vi "Name.vi"(8 "error in (no error)":errorcluster, 11 "object in":refnum<class "execute_request Message.lvclass">) -> (0 "error out":errorcluster, 2 "Name":string, 3 "object out":refnum<class "execute_request Message.lvclass">)   [LabVIEW 2018, in "ClientMessaging.lvlib" / "execute_request Message.lvclass"]
uses:
  execute_request Message.lvclass
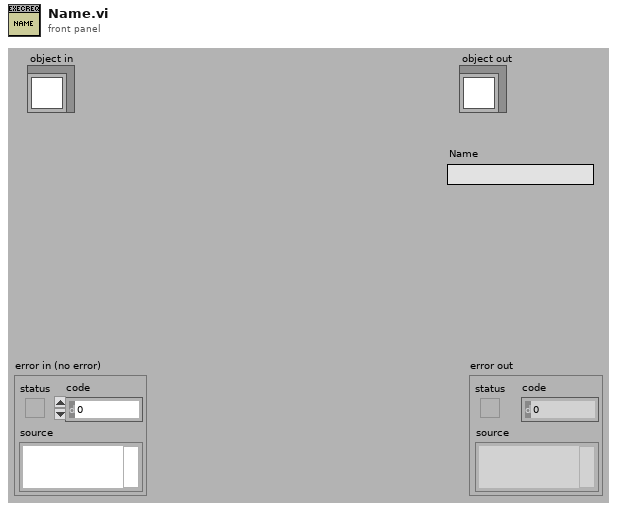
[diagram p1: front panel]
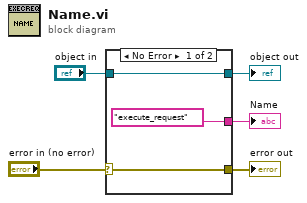
[diagram p0: block diagram]
diagram:
  n1 = case shown="No Error" "error in (no error)" {
    selector: "error in (no error)" -> [w7 w10]
    tunnel: [w7 w10] -> w4
    tunnel: [w8 w9] -> w2
    tunnel: "object in" -> [w8 w9]
    tunnel: ["execute_request" _] -> w1
    frame No Error {
    }
    frame Error {
    }
  }
  "error out" <- w4
  "object out" <- w2
  "Name" <- w1
